vi "sxpar.vi"(1 "Param":string, 2 "Array":string[](array[string])) -> (0 "Value":string)   [LabVIEW 2019]
panel:
  out "index of element":i32
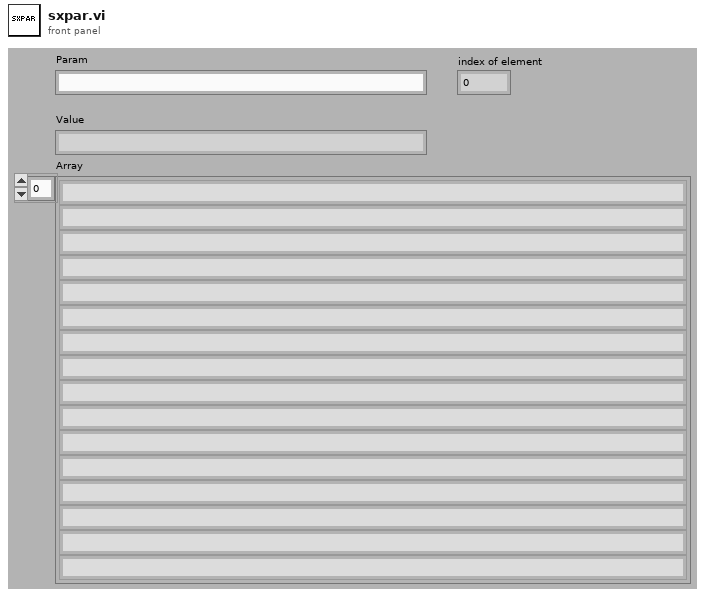
[diagram p1: front panel]
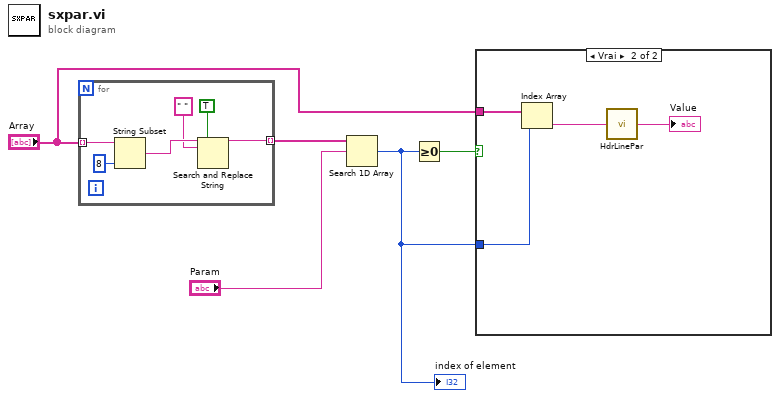
[diagram p0: block diagram]
diagram:
  n1 = for {
    tunnel: "Array" -> [w11] mode=indexing
    tunnel: [w7] -> w2 mode=indexing
    n2 = String Subset(string=w11, length (rest)=8 ("length (rest)")) -> (substring=w9:string)  [unwired: 1 in]
    n3 = Search and Replace String(replace all?=TRUE ("replace all? (F)"), input string=w9, search string=" ") -> (result string=w7:string)  [unwired: 5 in, 3 out]
  }
  n4 = Search 1D Array(1D array=w2, element="Param") -> (index of element=w3:i32)  [unwired: 1 in]
  "index of element" <- w3
  n5 = Greater Or Equal To 0?(x=w3) -> (x >= 0?=w4:bool)
  n6 = case shown="Vrai" w4 {
    tunnel: w3 -> [_ w14]
    tunnel: "Array" -> [_ w15]
    frame False {
    }
    frame True {
      n7 = Index Array(array=w15, index=w14) -> (element=w13:string)
      n8 = call "HdrLinePar.vi"("String"=w13) -> ("Valeur"=→"Value":string)  [unwired: 2 out]
    }
  }
